vi "Loop_SM.vi"() -> ()   [LabVIEW 2017, in "Intake.lvlib"]
uses:
  Intake.lvlib
  TypeDefs/Cluster_SRX Status No Encoder.ctl
  Cluster_Cmd to SM Data.ctl
  Enum_SM Cmd Select.ctl
  ENUM_State.ctl
  ENUM_Action.ctl
  Globals/Global_STOP.vi
  Global_CMD to SM Data.vi
  Global_HW_Status.vi
  Global_SM to HW Data.vi
panel:
  out "Vbus OUT":dbl
  out "CMD_Intake":T1
  out "HW_Intake_Status":T3
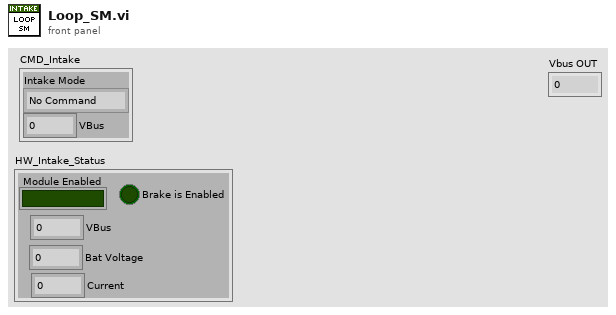
[diagram p1: front panel]
types:
  T1 = typedef "Intake.lvlib/Cluster_Cmd to SM Data.ctl" = cluster{"Intake Mode":T2, "VBus":dbl}
  T2 = typedef "Intake.lvlib/Enum_SM Cmd Select.ctl" = enum16{"No Command", "Manual", "Half Speed", "Full Speed", "Reverse", "Stop"}
  T3 = typedef "Cluster_SRX Status No Encoder.ctl" = cluster{"VBus ":dbl, "Module Enabled":bool, "Current":dbl, "Brake is Enabled":bool, "Bat Voltage":dbl}
  T4 = typedef "Intake.lvlib/ENUM_State.ctl" = enum16{"Startup", "Idle", "Auto", "Manual", "Shutdown"}
  T5 = typedef "Intake.lvlib/ENUM_Action.ctl" = enum16{"No Action", "Reset Time", "Stop", "Full Fwd", "Half Fwd", "Full Reverse", "Half Reverse", "Set Value"}
  T6 = cluster{"Actions":T5[], "State":T4, "Current Time":timestamp, "Start Time":timestamp, "Loop Time (ms)":u32, "CMD_Intake":T1, "HW_Status":T3, "Vbus OUT":dbl, "Full Fwd":dbl, "Half Fwd":dbl, "Full Reverse":dbl, "Half Reverse":dbl}
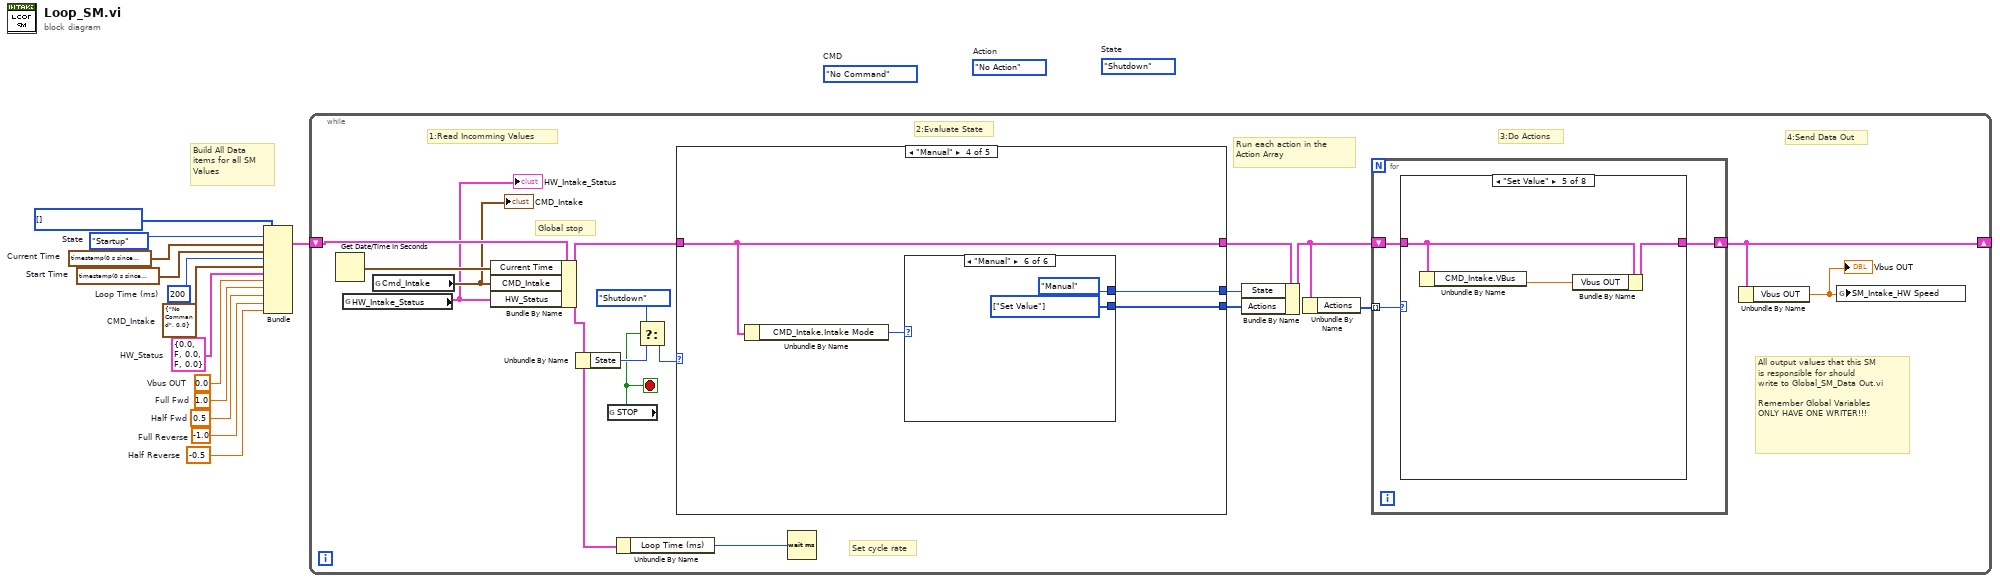
[diagram p0: block diagram]
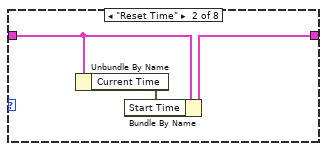
[diagram p3: hidden frame]
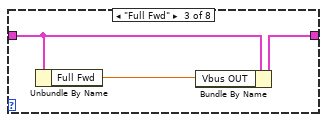
[diagram p4: hidden frame]
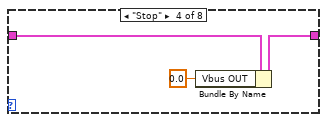
[diagram p5: hidden frame]
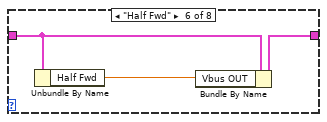
[diagram p6: hidden frame]
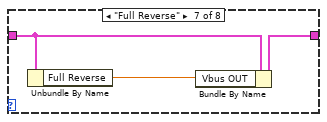
[diagram p7: hidden frame]
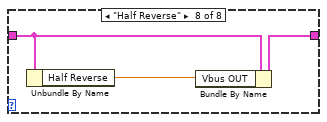
[diagram p8: hidden frame]
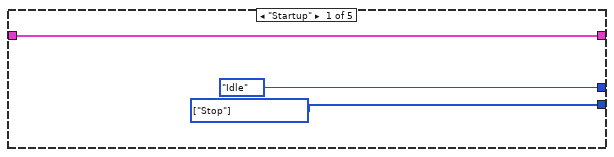
[diagram p9: hidden frame]
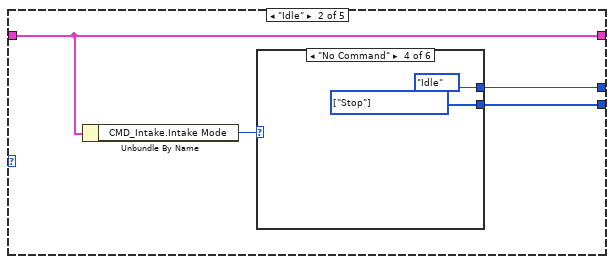
[diagram p10: hidden frame]
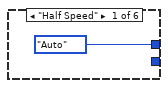
[diagram p11: hidden frame]
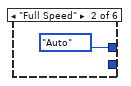
[diagram p12: hidden frame]
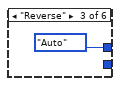
[diagram p13: hidden frame]
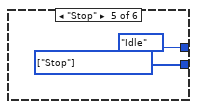
[diagram p14: hidden frame]
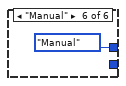
[diagram p15: hidden frame]
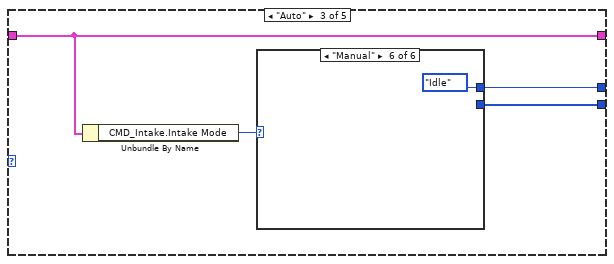
[diagram p16: hidden frame]
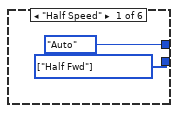
[diagram p17: hidden frame]
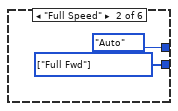
[diagram p18: hidden frame]
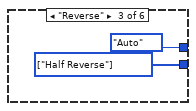
[diagram p19: hidden frame]
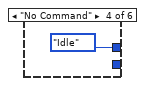
[diagram p20: hidden frame]
diagram:
  (unwired) ENUM_State."Shutdown"  # State
  (unwired) ENUM_Action."No Action"  # Action
  (unwired) Enum_SM_Cmd_Select."No Command"  # CMD
  w1 = -0.5  # Half Reverse
  w2 = -1.0  # Full Reverse
  w3 = 0.5  # Half Fwd
  w4 = 1.0  # Full Fwd
  w5 = 0.0  # Vbus OUT
  w6 = T3 {"VBus "=0.0, "Module Enabled"=FALSE, "Current"=0.0, "Brake is Enabled"=FALSE, "Bat Voltage"=0.0}  # HW_Status
  w7 = T1 {"Intake Mode"=enum."No Command", "VBus"=0.0}  # CMD_Intake
  w8 = u32 200  # Loop Time (ms)
  w9 = T5[] [] items=["No Action", "Reset Time", "Stop", "Full Fwd", "Half Fwd", "Full Reverse", "Half Reverse", "Set Value"] ("Actions")
  w10 = timestamp(0 s since 1904-01-01)  # Start Time
  w11 = timestamp(0 s since 1904-01-01)  # Current Time
  w12 = ENUM_State."Startup"  # State
  # "Build All Data items for all SM Values"
  n1 = Bundle("Actions"=w9, "State"=w12, "Current Time"=w11, "Start Time"=w10, "Loop Time (ms)"=w8, "CMD_Intake"=w7, "HW_Status"=w6, "Vbus OUT"=w5, "Full Fwd"=w4, "Half Fwd"=w3, "Full Reverse"=w2, "Half Reverse"=w1) -> (w13:T6)  [unwired: 1 in]
  n2 = while {
    shift-right: [w20] -> _
    shift-left: w13 -> [w29]
    stop <- w17 stop-if-true
    # "Set cycle rate"
    # "All output values that this SM\nis responsible for should\nwrite to Global_SM_Data Out.vi\n\nRemember Global Variables\nONLY HAVE ONE WRITER!!!"
    # "Run each action in the Action Array"
    # "1:Read Incomming Values"
    # "2:Evaluate State"
    # "3:Do Actions"
    # "4:Send Data Out"
    # "Global stop"
    n3 = Get Date/Time In Seconds() -> (seconds since 1Jan1904=w28:timestamp)
    n4 = global read "Global_HW_Status.vi" "HW_Intake_Status"() -> (w14:T3)
    "HW_Intake_Status" <- w14
    n5 = global read "Global_CMD to SM Data.vi" "Cmd_Intake"() -> (w15:T1)
    "CMD_Intake" <- w15
    n6 = Bundle By Name(cluster=w29, "Current Time"=w28, "CMD_Intake"=w15, "HW_Status"=w14) -> (w18:T6)
    n7 = Unbundle By Name(w18) -> ("State"=w22:T4)
    n8 = global read "Global_Stop.vi" "STOP"() -> (w17:bool)
    n9 = Unbundle By Name(w18) -> ("Loop Time (ms)"=w19:u32)
    n10 = Select(t=ENUM_State."Shutdown" ("State"), s=w17, f=w22) -> (s? t:f=w21:T4)
    n11 = case shown="\"Manual\"" w21 {
      tunnel: w18 -> [w58 w60 w72 w86 w98]
      tunnel: [w58 w60 w72 w86 w98] -> w26
      tunnel: [ENUM_State."Idle" ("State") w61 w73 w87 ENUM_State."Shutdown" ("State")] -> w25
      tunnel: [w57 w59 w71 w85 w96] -> w24
      frame "Startup" {
        w57 = T5[] [enum."Stop"] items=["No Action", "Reset Time", "Stop", "Full Fwd", "Half Fwd", "Full Reverse", "Half Reverse", "Set Value"] ("Actions")
      }
      frame "Idle" {
        n12 = Unbundle By Name(w60) -> ("CMD_Intake.Intake Mode"=w62:T2)
        n13 = case shown="\"No Command\"" w62 {
          tunnel: [ENUM_State."Auto" ("State") ENUM_State."Auto" ("State") ENUM_State."Auto" ("State") ENUM_State."Idle" ("State") ENUM_State."Idle" ("State") ENUM_State."Manual" ("State")] -> w61
          tunnel: [_ _ _ w66 w68 _] -> w59
          frame "Half Speed" {
          }
          frame "Full Speed" {
          }
          frame "Reverse" {
          }
          frame "No Command" {
            w66 = T5[] [enum."Stop"] items=["No Action", "Reset Time", "Stop", "Full Fwd", "Half Fwd", "Full Reverse", "Half Reverse", "Set Value"] ("Actions")
          }
          frame "Stop" {
            w68 = T5[] [enum."Stop"] items=["No Action", "Reset Time", "Stop", "Full Fwd", "Half Fwd", "Full Reverse", "Half Reverse", "Set Value"] ("Actions")
          }
          frame "Manual" {
          }
        }
      }
      frame "Auto" {
        n14 = Unbundle By Name(w72) -> ("CMD_Intake.Intake Mode"=w74:T2)
        n15 = case shown="\"Manual\"" w74 {
          tunnel: [ENUM_State."Auto" ("State") ENUM_State."Auto" ("State") ENUM_State."Auto" ("State") ENUM_State."Idle" ("State") ENUM_State."Idle" ("State") ENUM_State."Idle" ("State")] -> w73
          tunnel: [w75 w77 w79 _ w82 _] -> w71
          frame "Half Speed" {
            w75 = T5[] [enum."Half Fwd"] items=["No Action", "Reset Time", "Stop", "Full Fwd", "Half Fwd", "Full Reverse", "Half Reverse", "Set Value"] ("Actions")
          }
          frame "Full Speed" {
            w77 = T5[] [enum."Full Fwd"] items=["No Action", "Reset Time", "Stop", "Full Fwd", "Half Fwd", "Full Reverse", "Half Reverse", "Set Value"] ("Actions")
          }
          frame "Reverse" {
            w79 = T5[] [enum."Half Reverse"] items=["No Action", "Reset Time", "Stop", "Full Fwd", "Half Fwd", "Full Reverse", "Half Reverse", "Set Value"] ("Actions")
          }
          frame "No Command" {
          }
          frame "Stop" {
            w82 = T5[] [enum."Stop"] items=["No Action", "Reset Time", "Stop", "Full Fwd", "Half Fwd", "Full Reverse", "Half Reverse", "Set Value"] ("Actions")
          }
          frame "Manual" {
          }
        }
      }
      frame "Manual" {
        n16 = Unbundle By Name(w86) -> ("CMD_Intake.Intake Mode"=w88:T2)
        n17 = case shown="\"Manual\"" w88 {
          tunnel: [ENUM_State."Auto" ("State") ENUM_State."Auto" ("State") ENUM_State."Auto" ("State") ENUM_State."Idle" ("State") ENUM_State."Idle" ("State") ENUM_State."Manual" ("State")] -> w87
          tunnel: [_ _ _ _ _ w94] -> w85
          frame "Half Speed" {
          }
          frame "Full Speed" {
          }
          frame "Reverse" {
          }
          frame "No Command" {
          }
          frame "Stop" {
          }
          frame "Manual" {
            w94 = T5[] [enum."Set Value"] items=["No Action", "Reset Time", "Stop", "Full Fwd", "Half Fwd", "Full Reverse", "Half Reverse", "Set Value"] ("Actions")
          }
        }
      }
      frame "Shutdown" {
        w96 = T5[] [enum."Stop"] items=["No Action", "Reset Time", "Stop", "Full Fwd", "Half Fwd", "Full Reverse", "Half Reverse", "Set Value"] ("Actions")
      }
    }
    n18 = Wait (ms)(milliseconds to wait=w19) -> ()  [unwired: 1 out]
    n19 = Bundle By Name(cluster=w26, "State"=w25, "Actions"=w24) -> (w27:T6)
    n20 = Unbundle By Name(w27) -> ("Actions"=w30:T5[])
    n21 = for {
      tunnel: w30 -> [w33] mode=indexing
      shift-right: [w32] -> w20
      shift-left: w27 -> [w31]
      n22 = case shown="\"Set Value\"" w33 {
        tunnel: w31 -> [w34 w37 w39 w42 w45 w48 w51 w54]
        tunnel: [w34 w36 w40 w43 w46 w49 w52 w55] -> w32
        frame "No Action" {
        }
        frame "Reset Time" {
          n23 = Unbundle By Name(w37) -> ("Current Time"=w35:timestamp)
          n24 = Bundle By Name(cluster=w37, "Start Time"=w35) -> (w36:T6)
        }
        frame "Full Fwd" {
          n25 = Unbundle By Name(w39) -> ("Full Fwd"=w38:dbl)
          n26 = Bundle By Name(cluster=w39, "Vbus OUT"=w38) -> (w40:T6)
        }
        frame "Stop" {
          n27 = Bundle By Name(cluster=w42, "Vbus OUT"=0.0) -> (w43:T6)
        }
        frame "Set Value" {
          n28 = Unbundle By Name(w45) -> ("CMD_Intake.VBus"=w44:dbl)
          n29 = Bundle By Name(cluster=w45, "Vbus OUT"=w44) -> (w46:T6)
        }
        frame "Half Fwd" {
          n30 = Unbundle By Name(w48) -> ("Half Fwd"=w47:dbl)
          n31 = Bundle By Name(cluster=w48, "Vbus OUT"=w47) -> (w49:T6)
        }
        frame "Full Reverse" {
          n32 = Unbundle By Name(w51) -> ("Full Reverse"=w50:dbl)
          n33 = Bundle By Name(cluster=w51, "Vbus OUT"=w50) -> (w52:T6)
        }
        frame "Half Reverse" {
          n34 = Unbundle By Name(w54) -> ("Half Reverse"=w53:dbl)
          n35 = Bundle By Name(cluster=w54, "Vbus OUT"=w53) -> (w55:T6)
        }
      }
    }
    n36 = Unbundle By Name(w20) -> ("Vbus OUT"=w16:dbl)
    "Vbus OUT" <- w16
    n37 = global write "Global_SM to HW Data.vi" "SM_Intake_HW Speed"(w16) -> ()
  }
